vi "HEWH Determine Skip Draw and Purge.vi"(8 "Error In":errorcluster, 9 "Current Sequence Index":i32, 10 "PRAT/RLT Sequence":T2[](array[typedef]) {"Time" format="%<%H:%M:%S>t"}, 11 "Current Cond":T1) -> (0 "Error Out":errorcluster, 3 "Skip Draw And Purge":bool)   [LabVIEW 2016]
uses:
  Type Definitions/PRAT Test.ctl
  Utility/Save File/File Setup (Public)/Type Definition/Save File HEWH Heating Control Mode.ctl
  Type Definitions/Terminate Draw Conditions.ctl
  Type Definitions/HEWH Start Conditions.ctl
  Type Definitions/Check Special Condtions.ctl
  Type Definitions/HEWH Special Condition Check.ctl
  Type Definitions/HEWH Draw Flag ENUM.ctl
  Utility/Save File/File Setup.lvlib
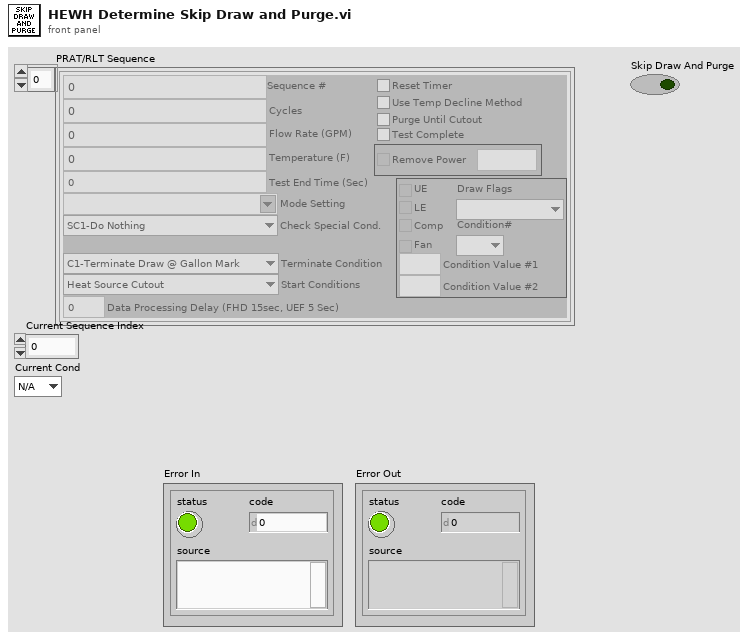
[diagram p1: front panel]
types:
  T1 = typedef "HEWH Special Condition Check.ctl" = enum16{"N/A", "C1", "C2", "Reset/Fail", "Skip Draw Sequence"}
  T2 = typedef "PRAT Test.ctl" = cluster{"Sequence #":dbl, "Cycles":i32, "Mode Setting":T3, "Flow Rate (GPM)":dbl, "Temperature (F)":dbl, "Reset Timer":bool, "Use Temp Decline Method":bool, "Terminate Condition":T4, "Condition Value #1":dbl, "UE":bool, "LE":bool, "Comp":bool, "Fan":bool, "Test End Time (Sec)":dbl, "Purge Until Cutout":bool, "Start Conditions":T5, "Condition Value #2":dbl, "Remove Power":bool, "Time":dbl, "Check Special Cond.":T6, "Condition#":T1, "Draw Flags":T7, "Data Processing Delay (FHD 15sec, UEF 5 Sec)":dbl, "Test Complete":bool}
  T3 = typedef "File Setup.lvlib/Save File HEWH Heating Control Mode.ctl" = string
  T4 = typedef "Terminate Draw Conditions.ctl" = enum16{"C1-Terminate Draw @ Gallon Mark", "C2-Special Last Draw (HU Test)", "C3-RTD Out <=", "C4-Mean Tank Temp <=", "C5-Decrease RTD Out (Deg F)", "C6-Time (Seconds)", "C7-Until Any Heat Source", "C8-Specific Heat Source", "C9-Do Nothing"}
  T5 = typedef "HEWH Start Conditions.ctl" = enum16{"Heat Source Cutout", "At Time (Seconds)", "Every X (Seconds)", "T2 >= X° Below Setpoint", "Seconds From Complete", "Wait for LE & Comp Cutout", "Wait for Comp Cutout", "Wait for LE Cutout", "Wait for UE Cutout"}
  T6 = typedef "Check Special Condtions.ctl" = enum16{"SC1-Do Nothing", "SC2-Check Heat Source (On-C2/Off-C1)", "SC3-Check Skip Condition", "SC4-Check Heat Source ON/Fail"}
  T7 = typedef "HEWH Draw Flag ENUM.ctl" = enum16{"N/A", "None(0)", "Sml(1)", "Med(2)", "SmlMed(3)", "Lrg(4)", "SmlLrg(5)", "MedLrg(6)", "SmlMedLrg(7)"}
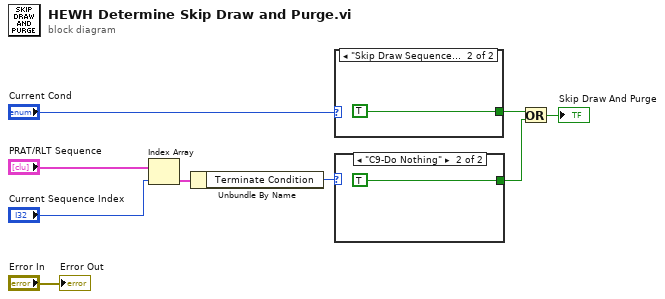
[diagram p0: block diagram]
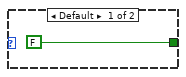
[diagram p2: hidden frame]
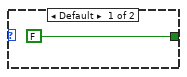
[diagram p3: hidden frame]
diagram:
  n1 = Index Array(array="PRAT/RLT Sequence", index="Current Sequence Index") -> (element=w6:T2)
  n2 = Unbundle By Name(w6) -> ("Terminate Condition"=w9:T4)
  n3 = case shown="\"Skip Draw Sequence\"" "Current Cond" {
    tunnel: [FALSE ("Skip Purge") TRUE ("Skip Purge")] -> w4
    frame Default {
    }
    frame "Skip Draw Sequence" {
    }
  }
  n4 = case shown="\"C9-Do Nothing\"" w9 {
    tunnel: [FALSE ("Skip Purge") TRUE ("Skip Purge")] -> w3
    frame Default {
    }
    frame "C9-Do Nothing" {
    }
  }
  n5 = Or(x=w4, y=w3) -> (x .or. y?=→"Skip Draw And Purge":bool)
  "Error Out" <- "Error In"
